vi "SEK2020v1SubVILerTamanhoTubo.vi"(1 "TamTubo":dbl) -> (0 "Numeric":i32)   [LabVIEW 2016]
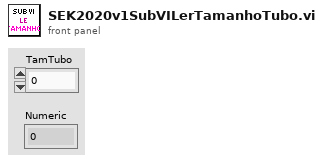
[diagram p1: front panel]
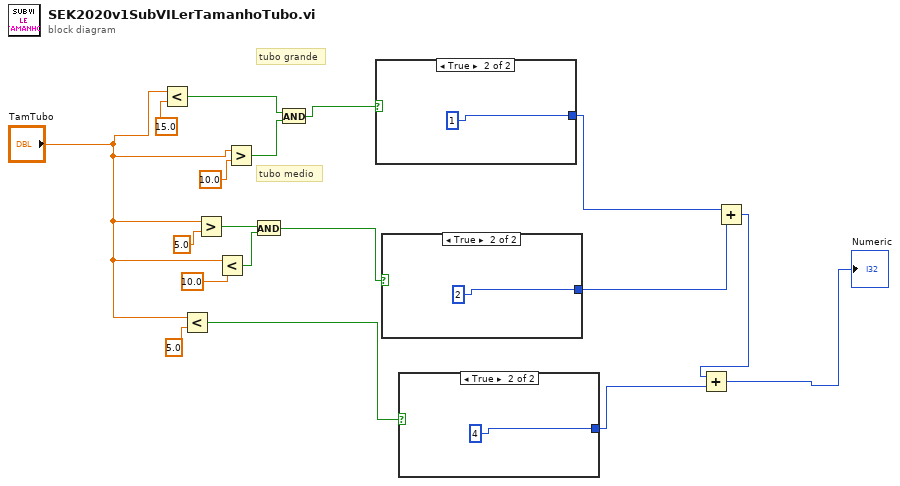
[diagram p0: block diagram]
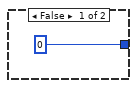
[diagram p2: hidden frame]
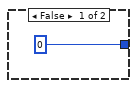
[diagram p3: hidden frame]
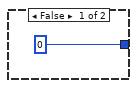
[diagram p4: hidden frame]
diagram:
  # "tubo medio"
  # "tubo grande"
  n1 = Less?(x="TamTubo", y=15.0) -> (x < y?=w15:bool)
  n2 = Less?(x="TamTubo", y=5.0) -> (x < y?=w6:bool)
  n3 = Greater?(x="TamTubo", y=5.0) -> (0:w12:bool)
  n4 = Less?(x="TamTubo", y=10.0) -> (x < y?=w11:bool)
  n5 = Greater?(x="TamTubo", y=10.0) -> (0:w14:bool)
  n6 = And(x=w12, y=w11) -> (x .and. y?=w7:bool)
  n7 = And(x=w15, y=w14) -> (x .and. y?=w8:bool)
  n8 = case shown="True" w8 {
    tunnel: [0 1] -> w5
    frame False {
    }
    frame True {
    }
  }
  n9 = case shown="True" w7 {
    tunnel: [0 2] -> w4
    frame False {
    }
    frame True {
    }
  }
  n10 = case shown="True" w6 {
    tunnel: [0 4] -> w3
    frame False {
    }
    frame True {
    }
  }
  n11 = Add(x=w5, y=w4) -> (x+y=w2:i32)
  n12 = Add(x=w2, y=w3) -> (x+y=→"Numeric":i32)
